vi "自动采样.vi"(7 "采样点数":i32=3, 8 "采样值":dbl[](array[numeric]), 9 "重新取值百分比":dbl=0.5, 10 "变异系数设定值":dbl=0.1, 11 "原始值":dbl) -> (0 "采样值输出":dbl[](array[numeric]), 1 "变异系数":dbl, 2 "mean":dbl caption="均值" format="%0.2f", 3 "取值输出":dbl, 5 "采样OK":bool)   [LabVIEW 2016, in "random number.lvlib"]
uses:
  random number.lvlib
  <vilib>/Analysis/baseanly.llb/Mean (DBL).vi
  <vilib>/Analysis/NI_AALBase.lvlib
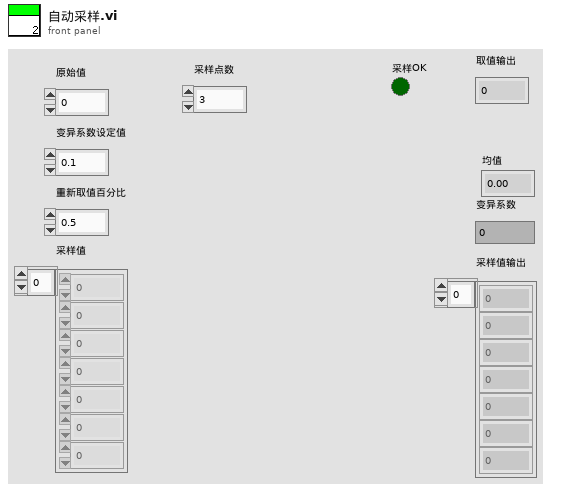
[diagram p1: front panel]
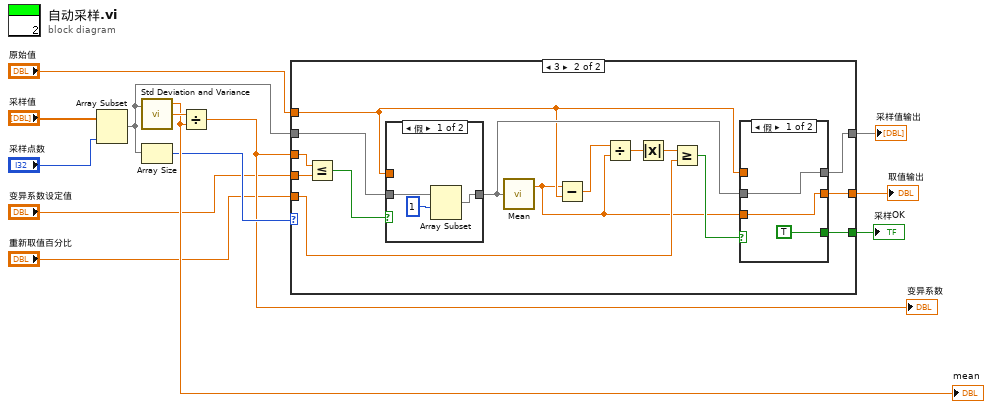
[diagram p0: block diagram]
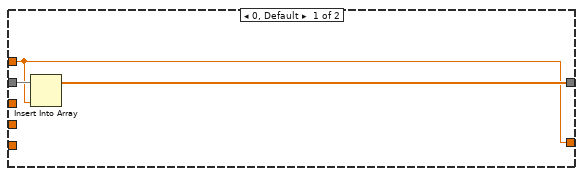
[diagram p2: hidden frame]
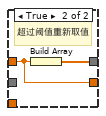
[diagram p3: hidden frame]
diagram:
  n1 = Array Subset(array="采样值", length="采样点数") -> (w8:dbl[])  [unwired: 1 in]
  n2 = call <vilib>:"Std Deviation and Variance.vi"("X"=w8) -> ("mean"=w12:dbl, "standard deviation"=w13:dbl)  [unwired: 1 in, 1 out]
  "mean" <- w12
  n3 = Array Size(array=w8) -> (size(s)=w9:i32)
  n4 = Divide(x=w13, y=w12) -> (x/y=w5:dbl)
  "变异系数" <- w5
  n5 = case shown="3" w9 {
    tunnel: w8 -> [w16 w31]
    tunnel: [w15 w21] -> w7
    tunnel: "原始值" -> [w14 w20]
    tunnel: w5 -> [_ w30]
    tunnel: "变异系数设定值" -> [_ w29]
    tunnel: [w14 w19] -> w3
    tunnel: "重新取值百分比" -> [_ w24]
    tunnel: [_ w17] -> w1
    frame 0, Default {
      n6 = Insert Into Array(array=w16, new element=w14) -> (w15:dbl[])  [unwired: 1 in]
    }
    frame 3 {
      n7 = Less Or Equal?(x=w30, y=w29) -> (x <= y?=w28:bool)
      n8 = case shown="假" w28 {
        tunnel: w31 -> [w39 w40]
        tunnel: [w38 w40] -> w22
        tunnel: w20 -> [_ _]
        frame False {
          n9 = Array Subset(array=w39, index=1 ("索引")) -> (w38:dbl[])  [unwired: 1 in]
        }
        frame True {
        }
      }
      n10 = call-poly <vilib>:"Mean.vi"("X"=w22) -> ("mean"=w18:dbl)  [unwired: 1 out]
      n11 = Subtract(x=w18, y=w20) -> (x-y=w27:dbl)
      n12 = Divide(x=w27, y=w18) -> (x/y=w26:dbl)
      n13 = Absolute Value(x=w26) -> (abs(x)=w25:dbl)
      n14 = Greater Or Equal?(x=w25, y=w24) -> (x >= y?=w23:bool)
      n15 = case shown="假" w23 {
        tunnel: w22 -> [w34 _]
        tunnel: [w34 w36] -> w21
        tunnel: w20 -> [_ w35]
        tunnel: [w33 w35] -> w19
        tunnel: w18 -> [w33 _]
        tunnel: [TRUE _] -> w17
        frame False {
        }
        frame True {
          # "超过阈值重新取值"
          n16 = Build Array(w35) -> (w36:dbl[])
        }
      }
    }
  }
  "取值输出" <- w3
  "采样值输出" <- w7
  "采样OK" <- w1
